vi "Read pyCmdFilePath.vi"(8 "error in (no error)":errorcluster, 11 "pyCode in":refnum<class "pyCode.lvclass">) -> (0 "error out":errorcluster, 2 "pyCmdFilePath":path, 3 "pyCode out":refnum<class "pyCode.lvclass">)   [LabVIEW 2018, in "pyCode.lvclass"]
uses:
  pyCode.lvclass
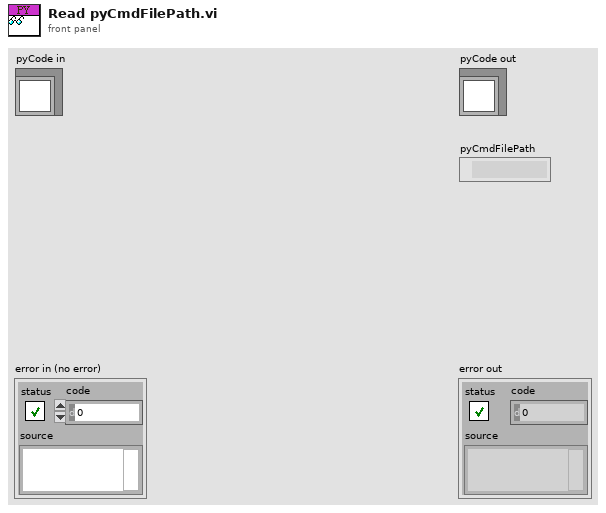
[diagram p1: front panel]
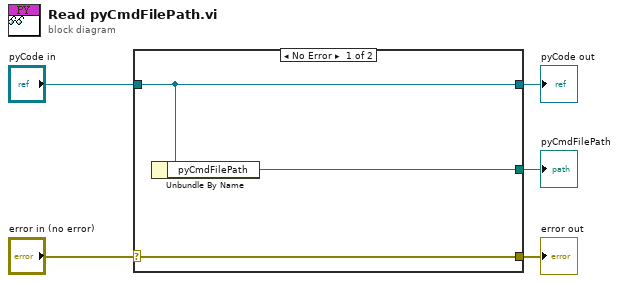
[diagram p0: block diagram]
diagram:
  n1 = case shown="No Error" "error in (no error)" {
    selector: "error in (no error)" -> [w8 w9]
    tunnel: [w8 w9] -> w4
    tunnel: [w7 w10] -> w2
    tunnel: "pyCode in" -> [w7 w10]
    tunnel: [w6 _] -> w1
    frame No Error {
      n2 = Unbundle By Name(w7) -> ("pyCmdFilePath"=w6:path)
    }
    frame Error {
    }
  }
  "error out" <- w4
  "pyCode out" <- w2
  "pyCmdFilePath" <- w1
